vi "Alarma_Modulacion_Frecuencia_G1.vi"(6 "# iteration":i32, 7 "ID_EQUIPO":i32, 11 "Frecuencia":sgl) -> (3 "Mod_Frec out":T1)   [LabVIEW 2018]
panel:
  out "error out":errorcluster
  in  "error in (no error)":errorcluster
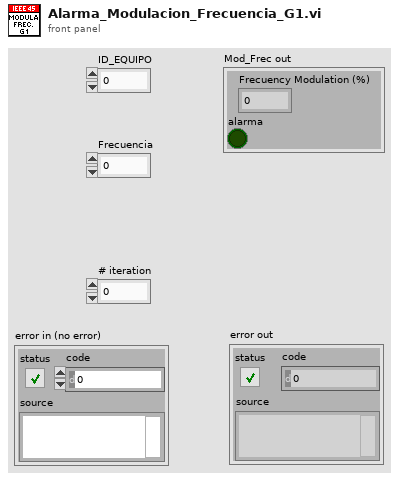
[diagram p1: front panel]
types:
  T1 = cluster{"Frecuency Modulation (%)":sgl, "alarma":bool}
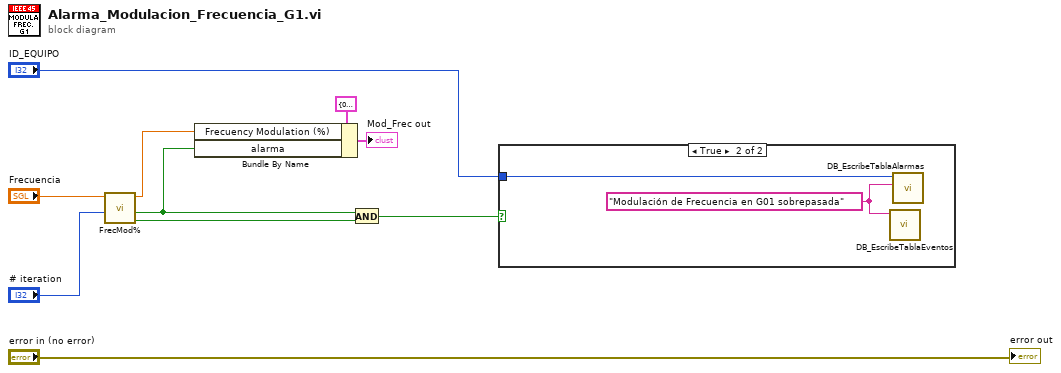
[diagram p0: block diagram]
diagram:
  n1 = call "FrecMod%.vi"("iteracion"="# iteration", "Frec Input"="Frecuencia") -> ("cada 10 seg"=w9:bool, "alarma"=w2:bool, "Frecuency Modulation (%)"=w3:sgl)  [unwired: 7 in]
  n2 = Bundle By Name(cluster=T1 {"Frecuency Modulation (%)"=0.0, "alarma"=FALSE}, "Frecuency Modulation (%)"=w3, "alarma"=w2) -> (→"Mod_Frec out":T1)
  n3 = And(x=w2, y=w9) -> (x .and. y?=w8:bool)
  n4 = case shown="True" w8 {
    tunnel: "ID_EQUIPO" -> [_ w12]
    frame False {
    }
    frame True {
      w11 = "Modulación de Frecuencia en G01 sobrepasada" ("MOTIVO")
      n5 = call "DB_EscribeTablaEventos.vi"("DESCRIPCION"=w11) -> ()  [unwired: 10 in, 1 out]
      n6 = call "DB_EscribeTablaAlarmas.vi"("MOTIVO"=w11, "ID_EQUIPO"=w12) -> ()  [unwired: 9 in, 1 out]
    }
  }
  "error out" <- "error in (no error)"
